vi "Read.vi"(8 "error in (no error)":errorcluster, 11 "PCANUSB in":refnum<class "PCANUSB.lvclass">) -> (0 "error out":errorcluster, 1 "Data":u8[](array[numeric]) format="%x", 2 "ID":u32 format="%x", 3 "PCANUSB out":refnum<class "PCANUSB.lvclass">, 4 "rcv queue empty":bool, 5 "CAN_Message out":T1 {"MSG type" format="%x"; "ID" format="%.0x"})   [LabVIEW 2024, in "PCANUSB.lvclass"]
uses:
  PCANUSB.lvclass
  PCANUSB.lvclass/PCANUSB.ctl
  PCAN/CAN Communication.llb/CAN MSG Cluster.ctl
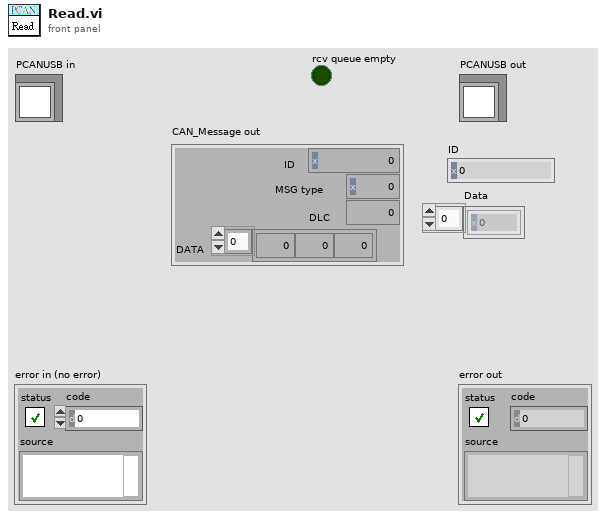
[diagram p1: front panel]
types:
  T1 = typedef "CAN MSG Cluster.ctl" = cluster{"ID":u32, "MSG type":u8, "DLC":u8, "DATA":u8[]}
  T2 = typedef "TPCANHandle.ctl" = enum16{"PCAN_NONEBUS  0x000", "PCAN_ISABUS1  0x21", "PCAN_ISABUS2  0x22", "PCAN_ISABUS3  0x23", "PCAN_ISABUS4  0x24", "PCAN_ISABUS5  0x25", "PCAN_ISABUS6  0x26", "PCAN_ISABUS7  0x27", "PCAN_ISABUS8  0x28", "PCAN_DNGBUS1  0x31", "PCAN_PCIBUS1  0x41", "PCAN_PCIBUS1  0x42", "PCAN_PCIBUS1  0x43", "PCAN_PCIBUS1  0x44", "PCAN_PCIBUS1  0x45", "PCAN_PCIBUS1  0x46", "PCAN_PCIBUS1  0x47", "PCAN_PCIBUS1  0x48", "PCAN_PCIBUS1  0x409", "PCAN_PCIBUS1  0x40A", "PCAN_PCIBUS1  0x40B", "PCAN_PCIBUS1  0x40C", "PCAN_PCIBUS1  0x40D", "PCAN_PCIBUS1  0x40E", "PCAN_PCIBUS1  0x40F", "PCAN_PCIBUS1  0x410", "PCAN_USBBUS1  0x51", "PCAN_USBBUS2  0x52", "PCAN_USBBUS3  0x53", "PCAN_USBBUS4  0x54", "PCAN_USBBUS5  0x55", "PCAN_USBBUS6  0x56", "PCAN_USBBUS7  0x57", "PCAN_USBBUS8  0x58", "PCAN_USBBUS9  0x509", "PCAN_USBBUS10  0x50A", "PCAN_USBBUS11  0x50B", "PCAN_USBBUS12  0x50C", "PCAN_USBBUS13  0x50D", "PCAN_USBBUS14  0x50E", "PCAN_USBBUS15  0x50F", "PCAN_USBBUS16  0x510", "PCAN_PCCBUS1  0x61", "PCAN_PCCBUS2  0x62", "PCAN_LANBUS1  0x801", "PCAN_LANBUS2  0x802", "PCAN_LANBUS3  0x803", "PCAN_LANBUS4  0x804", "PCAN_LANBUS5  0x805", "PCAN_LANBUS6  0x806", "PCAN_LANBUS7  0x807", "PCAN_LANBUS8  0x808", "PCAN_LANBUS9  0x809", "PCAN_LANBUS10  0x80A", "PCAN_LANBUS11  0x80B", "PCAN_LANBUS12  0x80C", "PCAN_LANBUS13  0x80D", "PCAN_LANBUS14  0x80E", "PCAN_LANBUS15  0x80F", "PCAN_LANBUS16  0x810"}
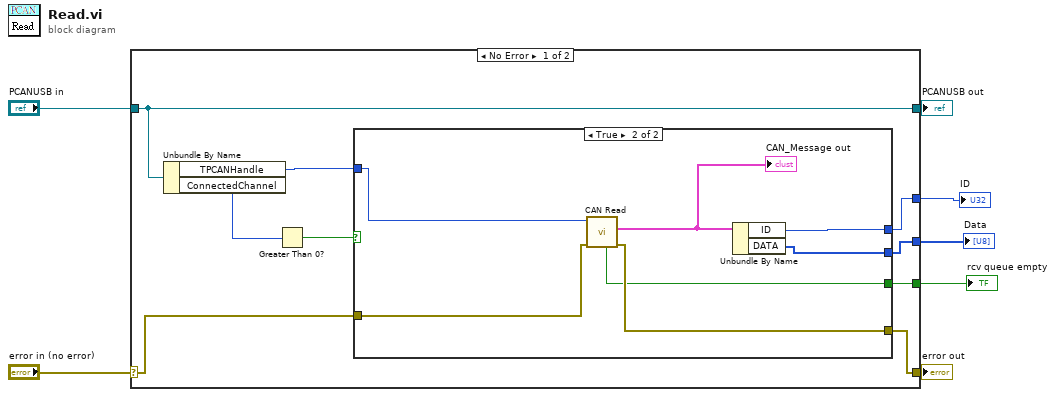
[diagram p0: block diagram]
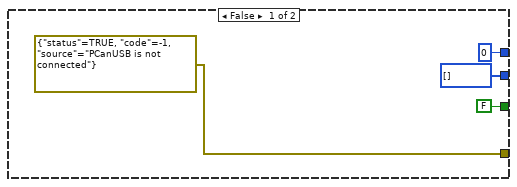
[diagram p2: hidden frame]
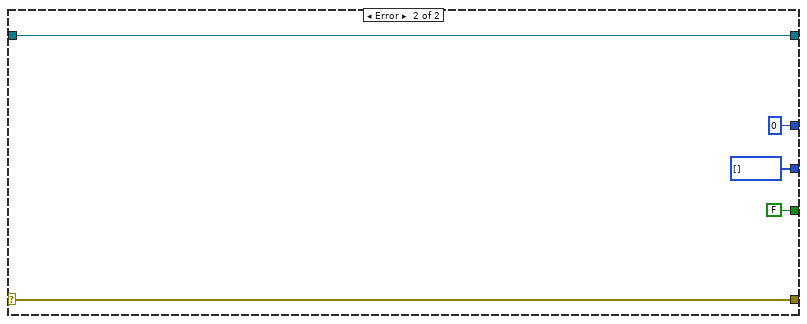
[diagram p3: hidden frame]
diagram:
  n1 = case shown="No Error" "error in (no error)" {
    selector: "error in (no error)" -> [w12 w32]
    tunnel: [w11 w32] -> w6
    tunnel: [w16 w31] -> w4
    tunnel: "PCANUSB in" -> [w16 w31]
    tunnel: [w10 u32 0 ("ID")] -> w3
    tunnel: [w9 u8[] [] ("DATA")] -> w2
    tunnel: [w8 FALSE ("rcv queue empty")] -> w1
    frame No Error {
      n2 = Unbundle By Name(w16) -> ("TPCANHandle"=w14:T2, "ConnectedChannel"=w13:u8)
      n3 = Greater Than 0?(x=w13) -> (x > 0?=w15:bool)
      n4 = case shown="True" w15 {
        tunnel: w14 -> [_ w21]
        tunnel: w12 -> [_ w27]
        tunnel: [errorcluster {"status"=TRUE, "code"=-1, "source"="PCanUSB is not connected"} ("error constant") w26] -> w11
        tunnel: [u32 0 ("ID") w24] -> w10
        tunnel: [u8[] [] ("DATA") w23] -> w9
        tunnel: [FALSE ("rcv queue empty") w22] -> w8
        frame False {
        }
        frame True {
          n5 = call "CAN Read.vi"("error in (no error)"=w27, "TPCANHandle"=w21) -> ("error out"=w26:errorcluster, "CAN_Message out"=w25:T1, "rcv queue empty"=w22:bool)  [unwired: 5 in, 2 out]
          "CAN_Message out" <- w25
          n6 = Unbundle By Name(w25) -> ("ID"=w24:u32, "DATA"=w23:u8[])
        }
      }
    }
    frame Error {
    }
  }
  "error out" <- w6
  "PCANUSB out" <- w4
  "rcv queue empty" <- w1
  "ID" <- w3
  "Data" <- w2
